vi "refreshListBox.vi"(8 "error in (no error)":errorcluster, 10 "Listbox":refnum<vi>, 11 "ExperimentRunner in":refnum<class "ExperimentRunner.lvclass">) -> (0 "error out":errorcluster, 2 "Listbox out":refnum<vi>, 3 "ExperimentRunner out":refnum<class "ExperimentRunner.lvclass">)   [LabVIEW 2011, in "Views.lvlib" / "ExperimentControl.lvlib" / "ExperimentRunner.lvclass"]
uses:
  ExperimentRunner.lvclass
  ExperimentRunner.lvclass/ExperimentRunner.ctl
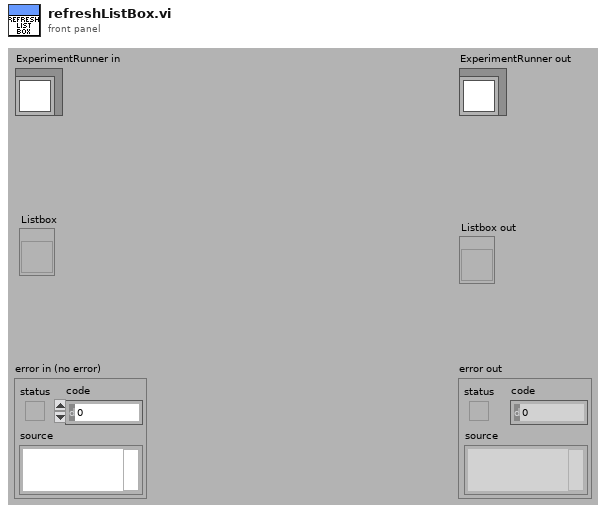
[diagram p1: front panel]
types:
  T1 = cluster{"CompilerPath":path, "CompilerString":string}[]
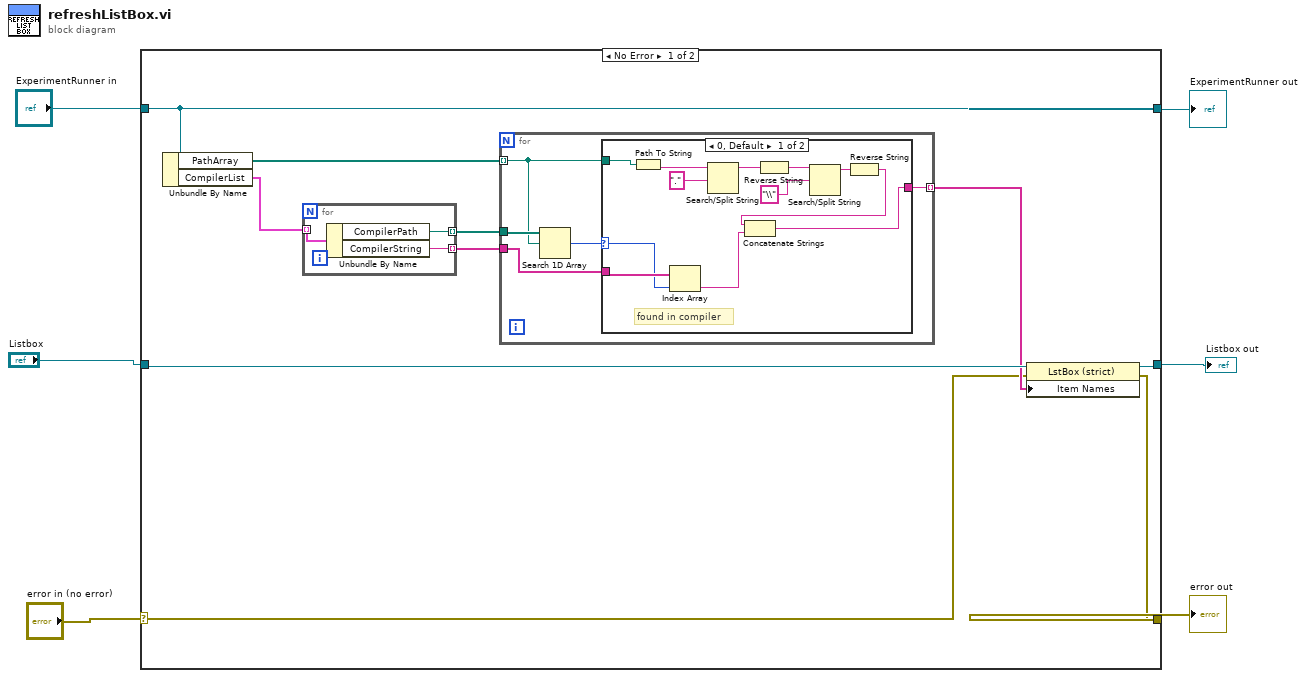
[diagram p0: block diagram]
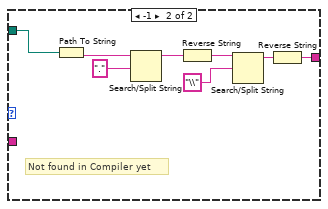
[diagram p2: hidden frame]
diagram:
  n1 = case shown="No Error" "error in (no error)" {
    selector: "error in (no error)" -> [w8 w47]
    tunnel: [w7 w47] -> w5
    tunnel: [w16 w46] -> w3
    tunnel: "ExperimentRunner in" -> [w16 w46]
    tunnel: "Listbox" -> [w10 w45]
    tunnel: [w11 w45] -> w1
    frame No Error {
      n2 = Unbundle By Name(w16) -> ("PathArray"=w15:path[], "CompilerList"=w14:T1)
      n3 = for {
        tunnel: w14 -> [w19] mode=indexing
        tunnel: [w18] -> w13 mode=indexing
        tunnel: [w17] -> w12 mode=indexing
        n4 = Unbundle By Name(w19) -> ("CompilerPath"=w18:path, "CompilerString"=w17:string)
      }
      n5 = for {
        tunnel: w15 -> [w22] mode=indexing
        tunnel: w13 -> [w24]
        tunnel: w12 -> [w21]
        tunnel: [w20] -> w9 mode=indexing
        n6 = Search 1D Array(1D array=w24, element=w22) -> (index of element=w23:i32)  [unwired: 1 in]
        n7 = case shown="0, Default" w23 {
          selector: w23 -> [w35 _]
          tunnel: w22 -> [w28 w38]
          tunnel: [w25 w37] -> w20
          tunnel: w21 -> [w36 _]
          frame 0, Default {
            # "found in compiler"
            n8 = Path To String(path=w28) -> (string=w34:string)
            n9 = Index Array(array=w36, index=w35) -> (element=w26:string)
            n10 = Search/Split String(string=w34, search string/char (-)=".") -> (substring before match=w32:string)  [unwired: 1 in, 2 out]
            n11 = Reverse String(1:w32) -> (0:w31:string)
            n12 = Search/Split String(string=w31, search string/char (-)="\\") -> (substring before match=w29:string)  [unwired: 1 in, 2 out]
            n13 = Reverse String(1:w29) -> (0:w27:string)
            n14 = Concatenate Strings(w27, w26) -> (w25:string)
          }
          frame -1 {
            # "Not found in Compiler yet"
            n15 = Path To String(path=w38) -> (string=w44:string)
            n16 = Search/Split String(string=w44, search string/char (-)=".") -> (substring before match=w42:string)  [unwired: 1 in, 2 out]
            n17 = Reverse String(1:w42) -> (0:w41:string)
            n18 = Search/Split String(string=w41, search string/char (-)="\\") -> (substring before match=w39:string)  [unwired: 1 in, 2 out]
            n19 = Reverse String(1:w39) -> (0:w37:string)
          }
        }
      }
      n20 = property class="LstBox (strict)"(reference=w10, error in=w8, "Item Names"=w9) -> (reference out=w11:refnum<vi>, error out=w7:errorcluster)
    }
    frame Error {
    }
  }
  "error out" <- w5
  "ExperimentRunner out" <- w3
  "Listbox out" <- w1
